vi "ECOG-Globals.vi"() -> ()   [LabVIEW 2020]
panel:
  in  "Version":string="1.0"
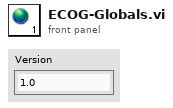
[diagram p1: front panel]
diagram:
